vi "MSEncoder Case-21-AuxScan.vi"(8 "error in (no error)":errorcluster, 9 "ParamValIn":variant, 11 "MSEncoder in":refnum<class "MSEncoder.lvclass">) -> (0 "error out":errorcluster, 3 "MSEncoder out":refnum<class "MSEncoder.lvclass">)   [LabVIEW 2018, in "MSEncoder.lvclass"]
uses:
  MSEncoder.lvclass
  Ctl/MSEditorParam auxScan.ctl
  PublicSubVI/Ctl/MathieuEqParam.ctl
  MSEncoder.lvclass/MSEncoder.ctl
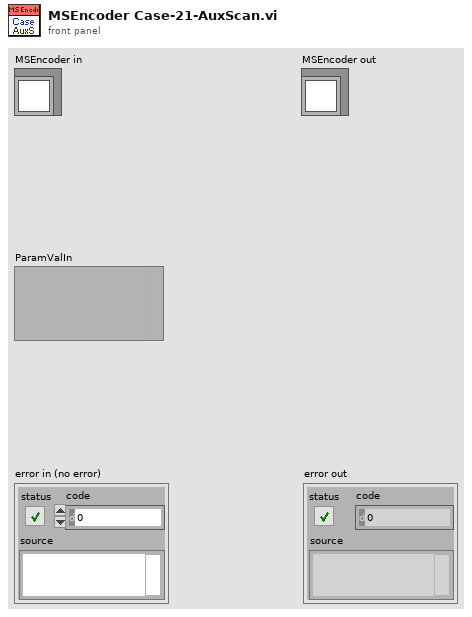
[diagram p1: front panel]
types:
  T1 = typedef "MSEditorParam auxScan.ctl" = cluster{"auxWfmType":u32, "auxStart":u32, "iauxCyc":ext, "auxCyc":ext[], "beta":ext[], "betaScale":ext, "auxAmp":ext[], "auxPulse1":ext[], "auxPulse2":ext[], "auxPulseAmp":ext[], "time":ext}
  T2 = typedef "MathieuEqParam.ctl" = cluster{"mz(Th)":ext, "Amp(V)":ext, "Freq(Hz)":ext, "Beta":ext, "r_0 (mm)":ext, "z_0 (mm)":ext}
  T3 = cluster{"Wfm type":u64, "Start conj #":u32, "TotalAuxCyc#":ext, "mz0":ext, "Scan rate":ext, "MathieuEqParame":T2, "Amp0":ext, "Amp ramp rate":ext, "Pulse1 Amp":ext, "Pulse2 Amp":ext, "Scan time":ext, "Beta scale":ext}
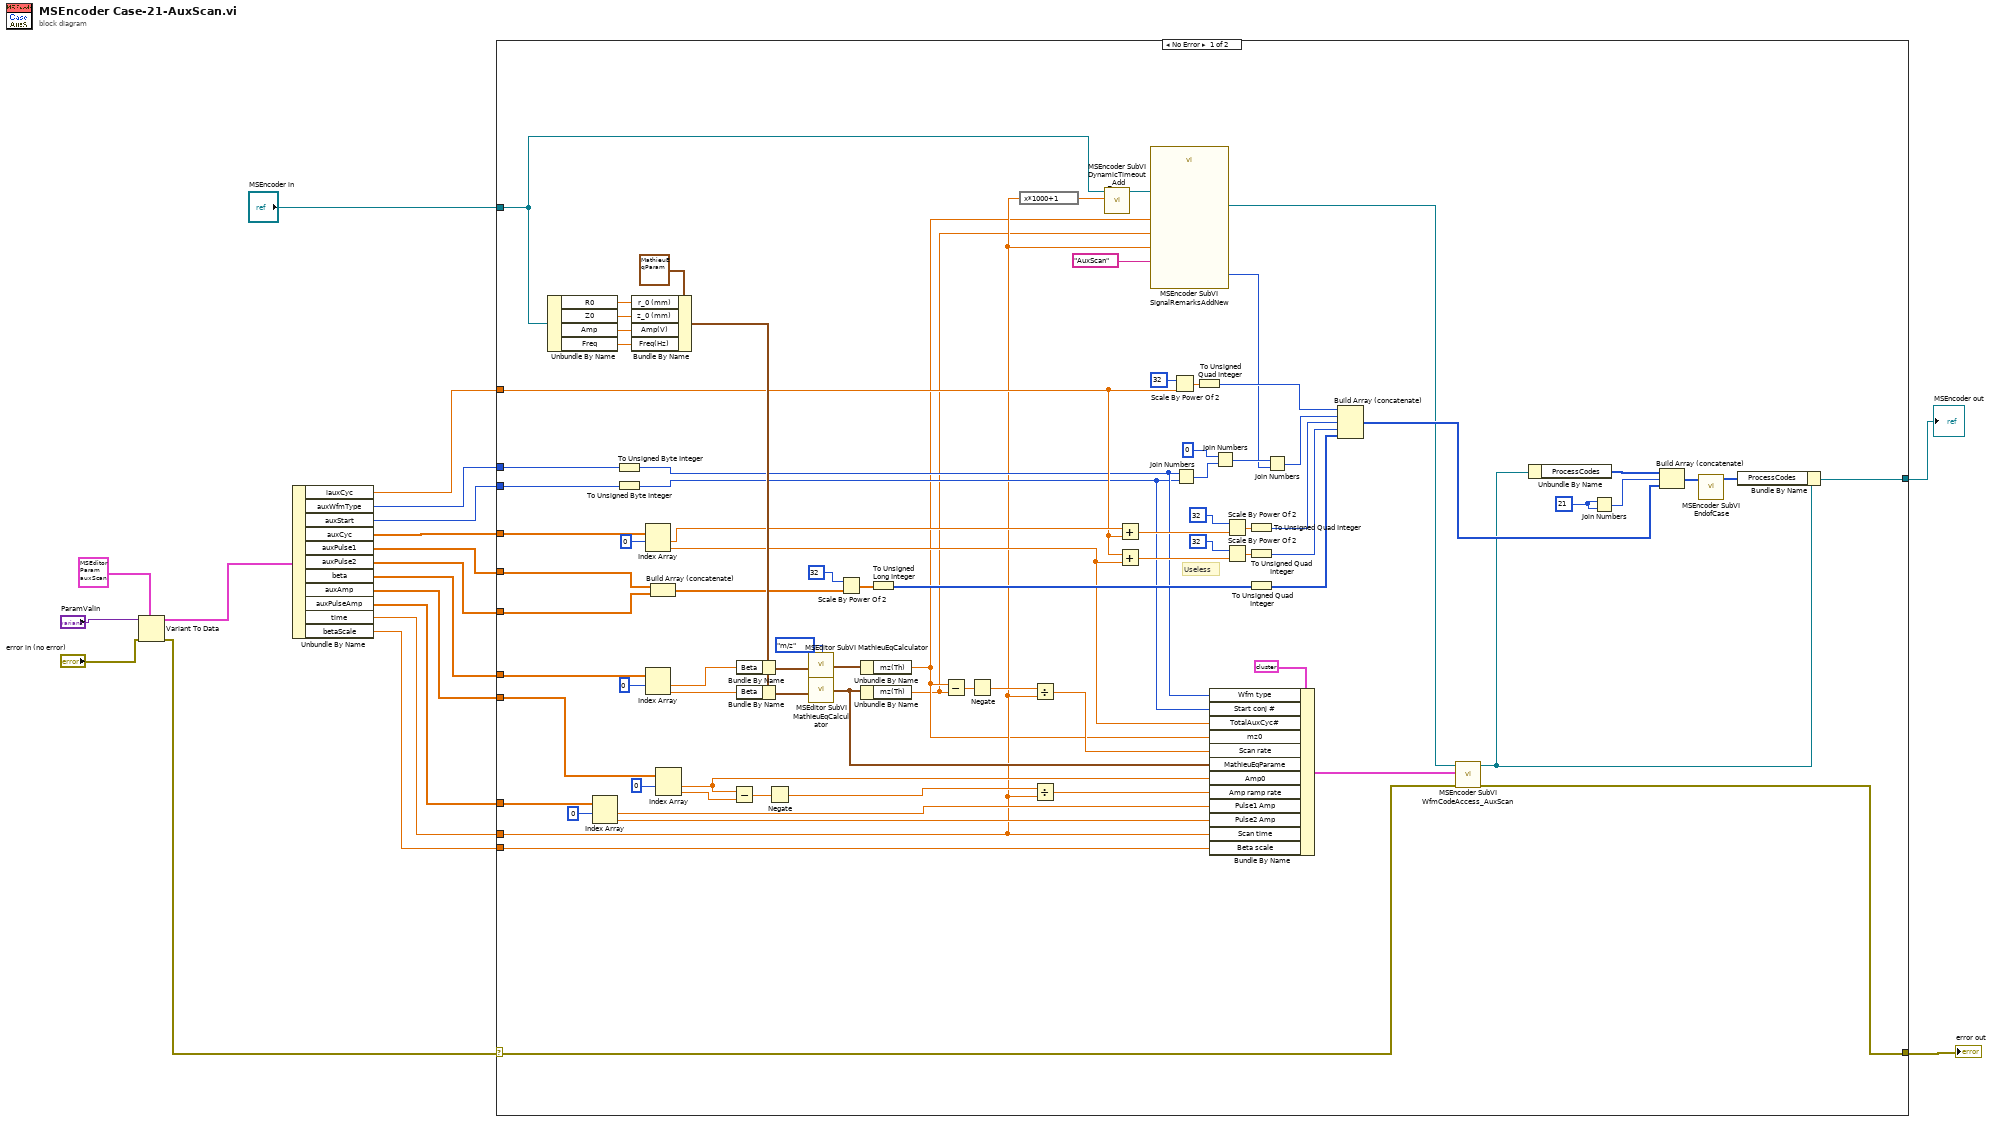
[diagram p0: block diagram]
diagram:
  n1 = Variant To Data(error in="error in (no error)", type=T1 {"auxWfmType"=0, "auxStart"=0, "iauxCyc"=0.0, "auxCyc"=[1.0, 1.0], "beta"=[0.1, 0.5], "betaScale"=1.0, "auxAmp"=[1.0, 1.0], "auxPulse1"=[0.0, 0.5], "auxPulse2"=[0.5, 1.0], "auxPulseAmp"=[1.0, -1.0], "time"=1.0} ("ParamValueType"), Variant="ParamValIn") -> (data=w3:T1, error out=w2:errorcluster)
  n2 = Unbundle By Name(w3) -> ("iauxCyc"=w18:ext, "auxWfmType"=w17:u32, "auxStart"=w16:u32, "auxCyc"=w15:ext[], "auxPulse1"=w14:ext[], "auxPulse2"=w13:ext[], "beta"=w12:ext[], "auxAmp"=w11:ext[], "auxPulseAmp"=w10:ext[], "time"=w9:ext, "betaScale"=w8:ext)
  n3 = case shown="No Error" w2 {
    selector: w2 -> [w37 w103]
    tunnel: "MSEncoder in" -> [w29 w102]
    tunnel: [w40 w103] -> w19
    tunnel: [w101 w102] -> w6
    tunnel: w18 -> [w59 _]
    tunnel: w17 -> [w58 _]
    tunnel: w16 -> [w57 _]
    tunnel: w15 -> [w56 _]
    tunnel: w14 -> [w55 _]
    tunnel: w13 -> [w54 _]
    tunnel: w12 -> [w53 _]
    tunnel: w11 -> [w52 _]
    tunnel: w10 -> [w51 _]
    tunnel: w9 -> [w26 _]
    tunnel: w8 -> [w41 _]
    frame No Error {
      w31 = u32 21
      w90 = enum16{"m/z", "Volt", "Freq", "Beta"}."m/z" ("Target (Freq)")
      # "Useless"
      n4 = Unbundle By Name(w29) -> ("R0"=w100:ext, "Z0"=w99:ext, "Amp"=w98:ext, "Freq"=w97:ext)
      n5 = Index Array(array=w51, index #1=0 ("index")) -> (element #1=w43:ext, element #2=w42:ext)  [unwired: 1 in]
      n6 = To Unsigned Byte Integer(number=w58) -> (unsigned 8bit integer=w49:u8)
      n7 = To Unsigned Byte Integer(number=w57) -> (unsigned 8bit integer=w48:u8)
      n8 = Bundle By Name(cluster=T2 {"mz(Th)"=0.0, "Amp(V)"=330.0, "Freq(Hz)"=0.0, "Beta"=1.0, "r_0 (mm)"=10.0, "z_0 (mm)"=7.0710678118654755} ("Parametres in"), "r_0 (mm)"=w100, "z_0 (mm)"=w99, "Amp(V)"=w98, "Freq(Hz)"=w97) -> (w95:T2)
      n9 = Index Array(array=w56, index #1=0 ("index")) -> (element #1=w71:ext, element #2=w47:ext)  [unwired: 1 in]
      n10 = Index Array(array=w53, index #1=0 ("index")) -> (element #1=w23:ext, element #2=w22:ext)  [unwired: 1 in]
      n11 = Build Array (concatenate)(w55, w54) -> (w63:ext[])
      n12 = Index Array(array=w52, index #1=0 ("index")) -> (element #1=w45:ext, element #2=w83:ext)  [unwired: 1 in]
      n13 = Subtract(x=w45, y=w83) -> (x-y=w85:ext)
      n14 = Bundle By Name(cluster=w95, "Beta"=w23) -> (w92:T2)
      n15 = Bundle By Name(cluster=w95, "Beta"=w22) -> (w91:T2)
      n16 = Negate(x=w85) -> (-x=w86:ext)
      n17 = call "MSEditor SubVI MathieuEqCalculator.vi"("Target (Freq)"=w90, "Parametres in"=w92) -> ("Parametres out"=w89:T2)  [unwired: 2 in]
      n18 = call "MSEditor SubVI MathieuEqCalculator.vi"("Target (Freq)"=w90, "Parametres in"=w91) -> ("Parametres out"=w46:T2)  [unwired: 2 in]
      n19 = Scale By Power Of 2(n=i16 32, x=w63) -> (x*2^n=w66:ext[])
      n20 = Unbundle By Name(w89) -> ("mz(Th)"=w21:ext)
      n21 = Unbundle By Name(w46) -> ("mz(Th)"=w20:ext)
      n22 = To Unsigned Long Integer(number=w66) -> (unsigned 32bit integer=w62:u32[])
      n23 = Subtract(x=w21, y=w20) -> (x-y=w88:ext)
      n24 = Negate(x=w88) -> (-x=w87:ext)
      n25 = expression code="x*1000+1"(w26) -> (w27:ext)
      n26 = Divide(x=w87, y=w26) -> (x/y=w35:ext)
      n27 = Divide(x=w86, y=w26) -> (x/y=w44:ext)
      n28 = call "MSEncoder SubVI DynamicTimeout_Add.vi"("Timeout_ms"=w27, "MSEncoder"=w29) -> ("MSEncoder"=w28:refnum<class "MSEncoder.lvclass">)  [unwired: 8 in, 1 out]
      n29 = Add(x=w71, y=w59) -> (x+y=w61:ext)
      n30 = Add(x=w59, y=w47) -> (x+y=w60:ext)
      n31 = call "MSEncoder SubVI SignalRemarksAddNew.vi"("Label"="AuxScan", "Scan time"=w26, "mz 1"=w20, "mz 0"=w21, "MSEncoder in"=w28) -> ("Len"=w24:u32, "MSEncoder out"=w36:refnum<class "MSEncoder.lvclass">)  [unwired: 5 in]
      n32 = Scale By Power Of 2(n=i16 32, x=w59) -> (x*2^n=w80:ext)
      n33 = Join Numbers(hi=w49, lo=w48) -> ((hi.lo)=w79:u16)
      n34 = To Unsigned Quad Integer(1:w80) -> (0:w75:u64)
      n35 = Bundle By Name(cluster=T3 {"Wfm type"=2, "Start conj #"=2, "TotalAuxCyc#"=3.0, "mz0"=880.97278970104787987, "Scan rate"=-33305.06819671684353, "MathieuEqParame"={"mz(Th)"=747.75251691418050576, "Amp(V)"=330.0, "Freq(Hz)"=199999.99552965164, "Beta"=0.8, "r_0 (mm)"=7.07106781187, "z_0 (mm)"=10.0}, "Amp0"=1.0, "Amp ramp rate"=-0.0, "Pulse1 Amp"=1.0, "Pulse2 Amp"=-1.0, "Scan time"=0.0039999999999999999998, "Beta scale"=1.0} ("AuxData"), "Wfm type"=w49, "Start conj #"=w48, "TotalAuxCyc#"=w47, "mz0"=w21, "Scan rate"=w35, "MathieuEqParame"=w46, "Amp0"=w45, "Amp ramp rate"=w44, "Pulse1 Amp"=w43, "Pulse2 Amp"=w42, "Scan time"=w26, "Beta scale"=w41) -> (w38:T3)
      n36 = Join Numbers(hi=u16 0, lo=w79) -> ((hi.lo)=w77:u32)
      n37 = Scale By Power Of 2(n=i16 32, x=w61) -> (x*2^n=w73:ext)
      n38 = Scale By Power Of 2(n=i16 32, x=w60) -> (x*2^n=w68:ext)
      n39 = To Unsigned Quad Integer(1:w73) -> (0:w70:u64)
      n40 = To Unsigned Quad Integer(1:w68) -> (0:w67:u64)
      n41 = To Unsigned Quad Integer(1:w62) -> (0:w65:u64[])
      n42 = Join Numbers(hi=w77, lo=w24) -> ((hi.lo)=w76:u64)
      n43 = Build Array (concatenate)(w75, w76, w70, w67, w65) -> (w64:u64[])
      n44 = call "MSEncoder SubVI WfmCodeAccess_AuxScan.vi"("error in"=w37, "Data in"=w38, "MSEncoder in"=w36) -> ("error out"=w40:errorcluster, "MSEncoder out"=w39:refnum<class "MSEncoder.lvclass">)  [unwired: 7 in]
      n45 = Unbundle By Name(w39) -> ("ProcessCodes"=w30:u64[])
      n46 = Join Numbers(hi=w31, lo=w31) -> ((hi.lo)=w34:u64)
      n47 = Build Array (concatenate)(w30, w34, w64) -> (w33:u64[])
      n48 = call "MSEncoder SubVI EndofCase.vi"("Case codes"=w33) -> ("Case codes with end"=w32:u64[])  [unwired: 9 in, 1 out]
      n49 = Bundle By Name(cluster=w39, "ProcessCodes"=w32) -> (w101:refnum<class "MSEncoder.lvclass">)
    }
    frame Error {
    }
  }
  "error out" <- w19
  "MSEncoder out" <- w6
